vi "AutoRangeMSO.vi"(0 "object in":refnum<class "AD2_SDK.lvclass">, 5 "error in (no error)":errorcluster) -> (14 "object out":refnum<class "AD2_SDK.lvclass">, 19 "error out":errorcluster)   [LabVIEW 2023, in "AD2_SDK.lvclass"]
uses:
  AD2_SDK.lvclass
  AD2_SDK.lvclass/AD2_SDK.ctl
  <vilib>/measure/matone.llb/Extract Single Tone Information 1 Chan.vi
  AD2_MSO_SDK_class/AD2_MSO_SDK.lvclass
  <vilib>/measure/NI_MAPro.lvlib
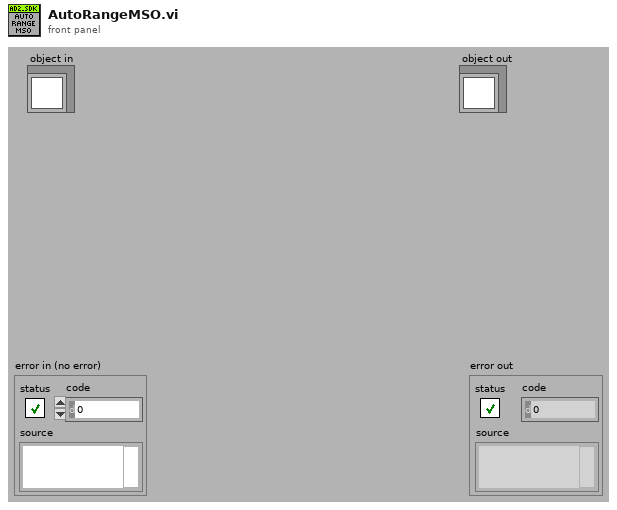
[diagram p1: front panel]
types:
  T1 = typedef "AD2_MSO_SDK.lvclass/MSOConfig.ctl" = cluster{"Timing":cluster{"Enable":bool, "Samples In":dbl, "Sample Rate":dbl, "Mode":enum16{"Single Sample", "Scanshift", "Multiple Samples", "Scan Screen"}}, "Trigger":cluster{"Hysteresis":dbl, "Trigger Level":dbl, "Trigger Condition":i32, "Trigger Type":i32, "Trigger Channel":i32, "secTimeout":dbl, "TrigrSrc":T2}, "Range Ch1":T3, "Range Ch 2":T3}
  T2 = typedef "AD2_MSO_SDK.lvclass/AD2TriggerSources.ctl" = enum8{"trigrsrcNone", "trigsrcPC", "trigsrcDetectorAnalogIn", "trigsrcDetectorDigitalIn", "trigsrcAnalogIn", "trigsrcDigitalIn", "trigsrcDigitalOut", "trigsrcAnalogOut1", "trigsrcAnalogOut2", "trigsrcAnalogOut3", "trigsrcAnalogOut4", "trigsrcExternal1", "trigsrcExternal2", "trigsrcExternal3", "trigsrcExternal4", ""}
  T3 = typedef "AD2_MSO_SDK.lvclass/MSORangeCh.ctl" = cluster{"idxChannel":i32, "voltOffset":dbl, "VoltsRange":u16}
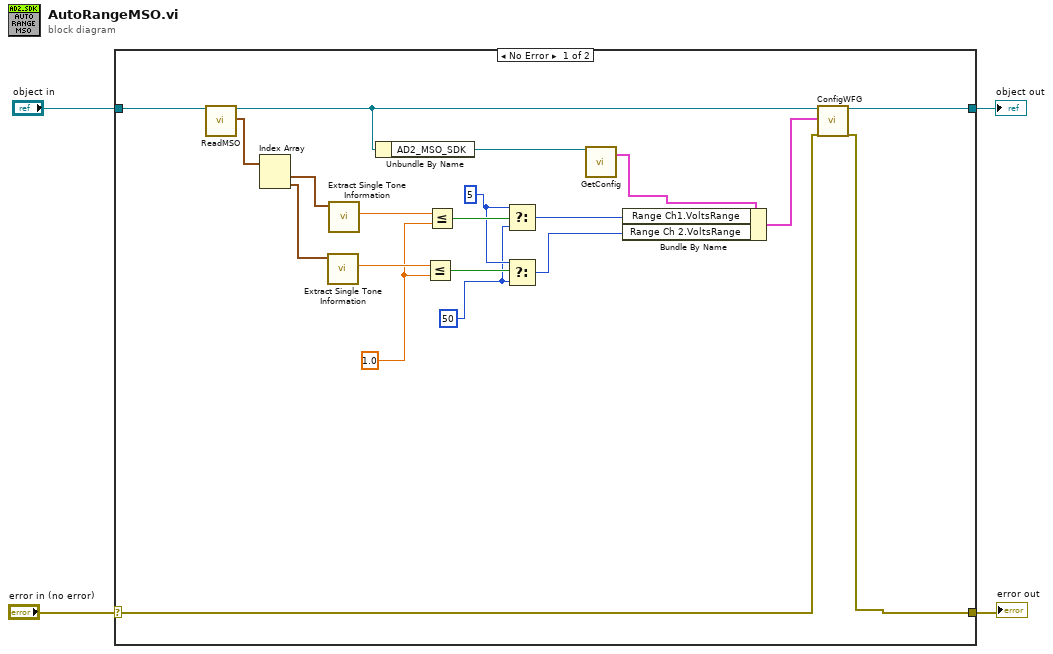
[diagram p0: block diagram]
diagram:
  n1 = case shown="No Error" "error in (no error)" {
    selector: "error in (no error)" -> [w8 w26]
    tunnel: [w7 w26] -> w3
    tunnel: [w21 w25] -> w1
    tunnel: "object in" -> [w24 w25]
    frame No Error {
      w13 = 1.0 ("y")
      w9 = u16 50 ("Range Ch1.VoltsRange")
      w15 = u16 5 ("Range Ch1.VoltsRange")
      n2 = call-dynamic "ReadMSO.vi"("object in"=w24) -> ("object out"=w22:refnum<class "AD2_SDK.lvclass">, "Channels array"=w5:waveform(dbl)[])  [unwired: 16 in, 1 out]
      n3 = Index Array(array=w5) -> (element #1=w20:waveform(dbl), element #2=w19:waveform(dbl))  [unwired: 2 in]
      n4 = call-poly <vilib>:"Extract Single Tone Information.vi"("time signal in"=w19) -> ("detected amplitude"=w17:dbl)  [unwired: 5 in, 5 out]
      n5 = call-poly <vilib>:"Extract Single Tone Information.vi"("time signal in"=w20) -> ("detected amplitude"=w18:dbl)  [unwired: 5 in, 5 out]
      n6 = Unbundle By Name(w22) -> ("AD2_MSO_SDK"=w23:refnum<class "AD2_MSO_SDK.lvclass">)
      n7 = Less Or Equal?(x=w17, y=w13) -> (x <= y?=w14:bool)
      n8 = Less Or Equal?(x=w18, y=w13) -> (x <= y?=w16:bool)
      n9 = Select(t=w15, s=w16, f=w9) -> (s? t:f=w12:u16)
      n10 = Select(t=w15, s=w14, f=w9) -> (s? t:f=w11:u16)
      n11 = call-dynamic "GetConfig.vi"("object in"=w23) -> ("Config"=w6:T1)  [unwired: 16 in, 2 out]
      n12 = Bundle By Name(cluster=w6, "Range Ch1.VoltsRange"=w12, "Range Ch 2.VoltsRange"=w11) -> (w10:T1)
      n13 = call-dynamic "ConfigWFG.vi"("object in"=w22, "Config(var)"=w10, "error in (no error)"=w8) -> ("object out"=w21:refnum<class "AD2_SDK.lvclass">, "error out"=w7:errorcluster)  [unwired: 15 in]
    }
    frame Error {
    }
  }
  "error out" <- w3
  "object out" <- w1
